vi "Init Msg Default.vi"() -> (2 "Msg":refnum<class "Msg.lvclass">)   [LabVIEW 2020, in "_Template.lvlib" / "Templates.lvlib" / "TEMPLATE jettl Msg.lvlib" / "TEMPLATE Msg.lvlib"]
uses:
  TEMPLATE Msg.lvlib
  jettl/jettl/Msg/Msg.lvclass
  TEMPLATE Msg/TEMPLATE Msg.lvclass
  C:/git/jettl/src/jettl/jettl/Msg/Msg.lvclass
panel:
  # "This front panel should not be manipulated."
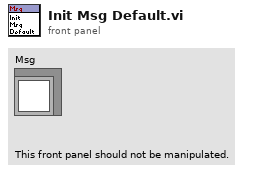
[diagram p1: front panel]
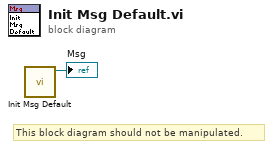
[diagram p0: block diagram]
diagram:
  # "This block diagram should not be manipulated."
  n1 = call "Init Msg Default.vi"() -> ("TEMPLATE Msg out"=→"Msg":refnum<class "TEMPLATE Msg.lvclass">)  [unwired: 11 in]
